vi "SBML_Mod_Def.vi"(8 "error in (no error)":errorcluster, 11 "Input SBML File":string) -> (0 "error out":errorcluster, 2 "Mod_Idx":i32[](array[numeric]), 3 "Mod_ID":string[](array[string]))   [LabVIEW 2014]
doc: "This VI extract the information of species present in SBML file. It takes the complete SBML file as input, and outputs: \nSp_Cnt --> How many species are there\nS_Id_Arr --> Array of species\nSp_Name --> Array containing the name of species\nSp_Init_Amnt --> Array containing the initial amount of species\n\nDesigned by HB\nhaba@dtu.dk"
panel:
  out "Mod_Idx":string[](array[string])
  out "Mod_Cnt":i32
  out "List of Mods":string
  # "Names"
  # "Initial Amount"
  # "ID"
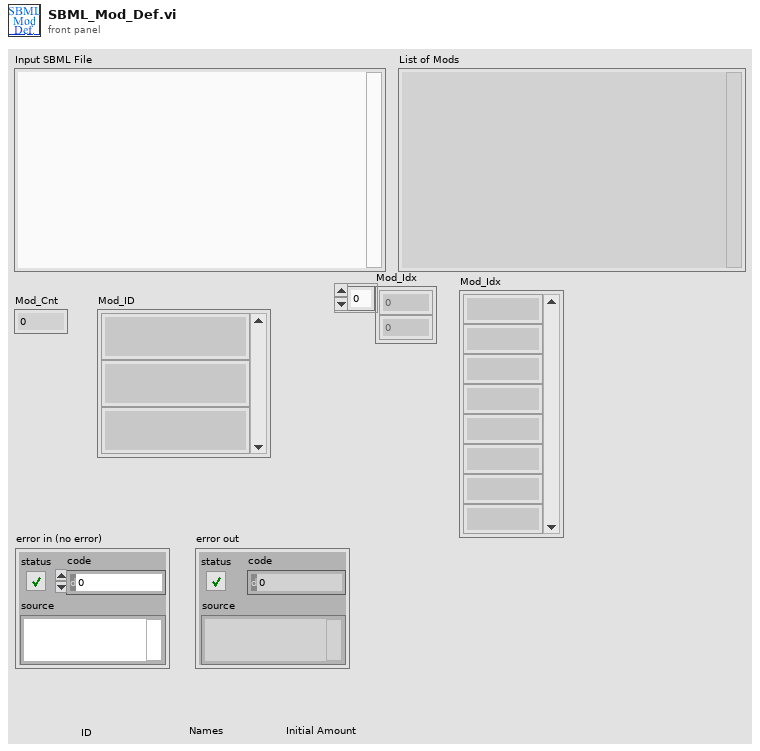
[diagram p1: front panel]
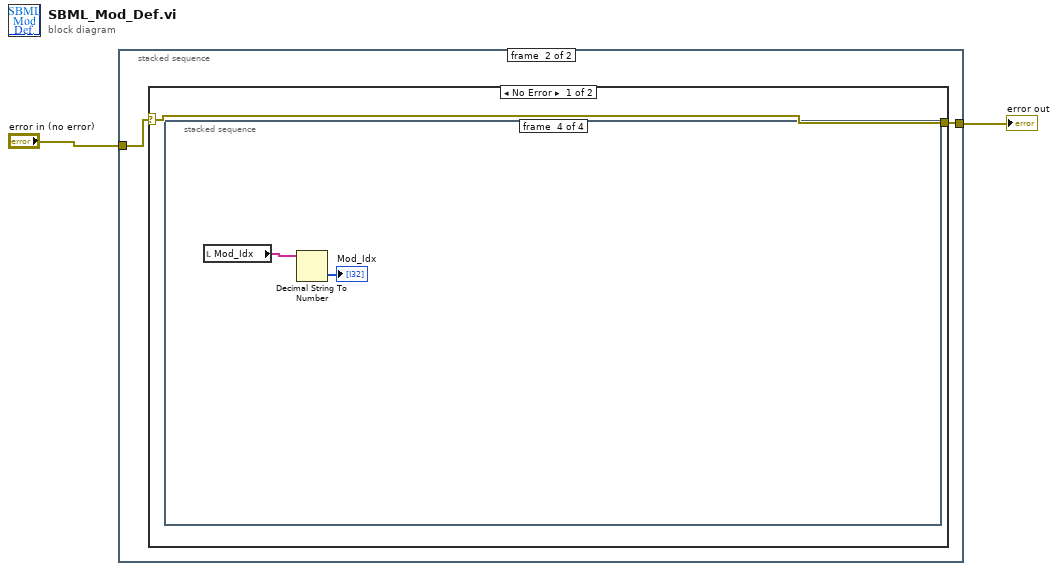
[diagram p0: block diagram]
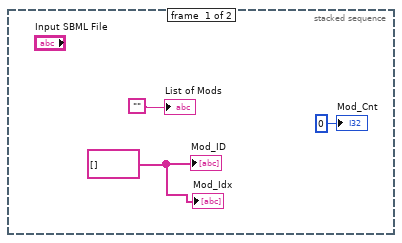
[diagram p2: hidden frame]
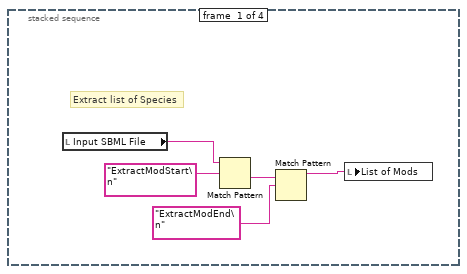
[diagram p3: hidden frame]
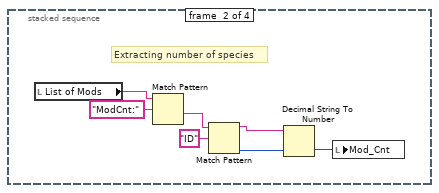
[diagram p4: hidden frame]
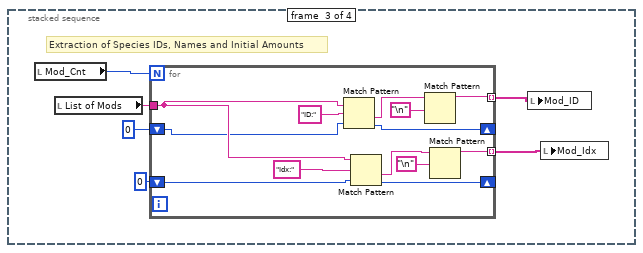
[diagram p5: hidden frame]
diagram:
  n1 = stacked-sequence {
    tunnel: "error in (no error)" -> [_ w6]
    tunnel: [_ w7] -> w1
    frame #0 {
      w3 = string[] [] ("Sp_Id_Arr")
      "List of Mods" <- "" ("Full SBML File")
      "Mod_Cnt" <- 0 ("Sp_cnt")
      "Mod_ID" <- w3
      "Mod_Idx" <- w3
    }
    frame #1 {
      n2 = case shown="No Error" w6 {
        selector: w6 -> [w8 w42]
        tunnel: [w8 w42] -> w7
        frame No Error {
          n3 = stacked-sequence {
            frame #0 {
              # "Extract list of Species"
              n4 = local read "Input SBML File"() -> (w10:string)
              n5 = Match Pattern(string=w10, regular expression="ExtractModStart\n") -> (after substring=w12:string)  [unwired: 1 in, 3 out]
              n6 = Match Pattern(string=w12, regular expression="ExtractModEnd\n") -> (before substring=w9:string)  [unwired: 1 in, 3 out]
              n7 = local write "List of Mods"(w9) -> ()
            }
            frame #1 {
              # "Extracting number of species"
              n8 = local read "List of Mods"() -> (w18:string)
              n9 = Match Pattern(string=w18, regular expression="ModCnt:") -> (after substring=w15:string)  [unwired: 1 in, 3 out]
              n10 = Match Pattern(string=w15, regular expression="ID") -> (before substring=w14:string, offset past match=w16:i32)  [unwired: 1 in, 2 out]
              n11 = Decimal String To Number(string=w14, default (0L)=w16) -> (number=w19:i32)  [unwired: 1 in, 1 out]
              n12 = local write "Mod_Cnt"(w19) -> ()
            }
            frame #2 {
              # "Extraction of Species IDs, Names and Initial Amounts"
              n13 = local read "Mod_Cnt"() -> (w24:i32)
              n14 = local read "List of Mods"() -> (w25:string)
              n15 = for {
                N: w24 -> [_]
                tunnel: w25 -> [w29]
                shift-right: [w27] -> _
                shift-left: 0 ("offset past match") -> [w28]
                tunnel: [w36] -> w23 mode=indexing
                shift-right: [w33] -> _
                shift-left: 0 ("offset past match") -> [w34]
                tunnel: [w35] -> w22 mode=indexing
                n16 = Match Pattern(string=w29, regular expression="ID:", offset (0)=w28) -> (after substring=w37:string, offset past match=w27:i32)  [unwired: 2 out]
                n17 = Match Pattern(string=w29, regular expression="Idx:", offset (0)=w34) -> (after substring=w30:string, offset past match=w33:i32)  [unwired: 2 out]
                n18 = Match Pattern(string=w37, regular expression="\n") -> (before substring=w36:string)  [unwired: 1 in, 3 out]
                n19 = Match Pattern(string=w30, regular expression="\n") -> (before substring=w35:string)  [unwired: 1 in, 3 out]
              }
              n20 = local write "Mod_ID"(w23) -> ()
              n21 = local write "Mod_Idx"(w22) -> ()
            }
            frame #3 {
              n22 = local read "Mod_Idx"() -> (w41:string[])
              n23 = Decimal String To Number(string=w41) -> (number=→"Mod_Idx":i32[])  [unwired: 2 in, 1 out]
            }
          }
        }
        frame Error {
        }
      }
    }
  }
  "error out" <- w1
